vi "Handle Request.vi"(8 "error in (no error)":errorcluster, 9 "Payload":string, 10 "Method":string, 11 "Child Class in":refnum<class "Instrument.lvclass">) -> (0 "error out":errorcluster, 2 "Response":string, 3 "Child Class out":refnum<class "Instrument.lvclass">)   [LabVIEW 2017, in "Instrument.lvlib" / "Instrument.lvclass"]
uses:
  Instrument.lvclass
  <vilib>/TSS/ACRObat Test Framework/Classes/Base Objects/Acrobat Base Object/Acrobat Base Object/Acrobat Base Object.lvclass
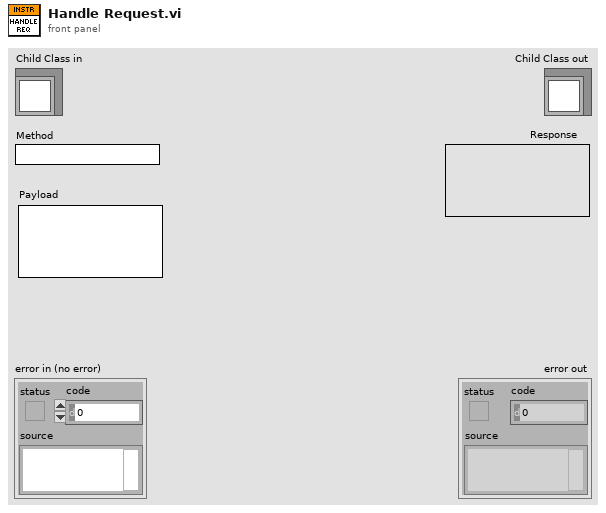
[diagram p1: front panel]
types:
  T1 = cluster{"Self-Test Result Code":i32, "Self-Test Result Message":string}
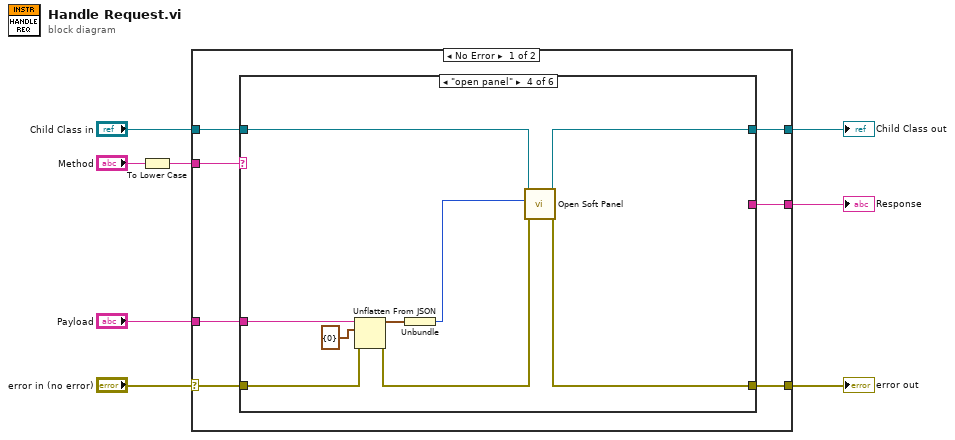
[diagram p0: block diagram]
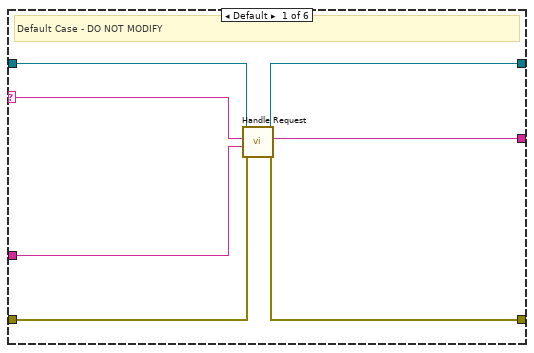
[diagram p2: hidden frame]
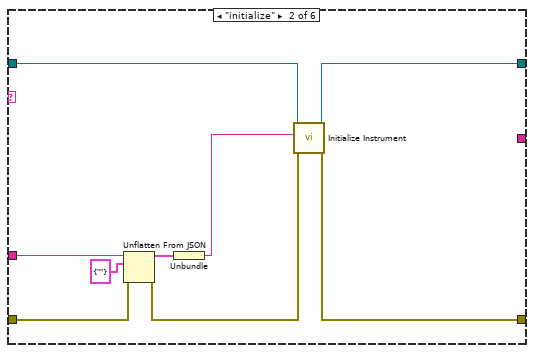
[diagram p3: hidden frame]
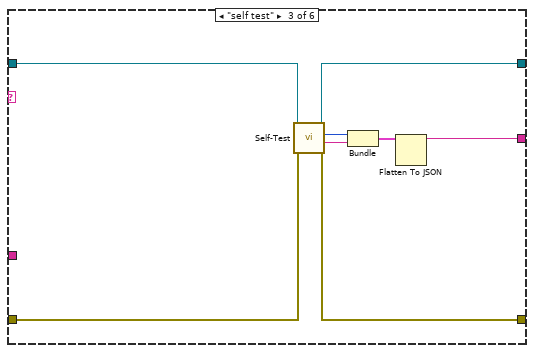
[diagram p4: hidden frame]
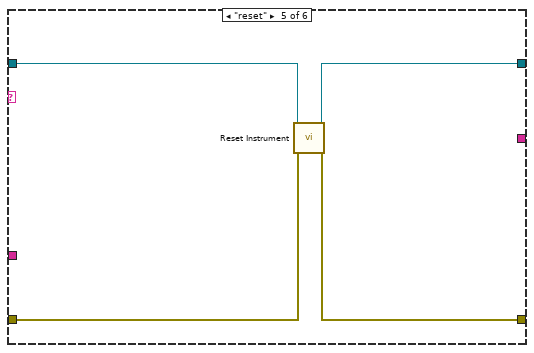
[diagram p5: hidden frame]
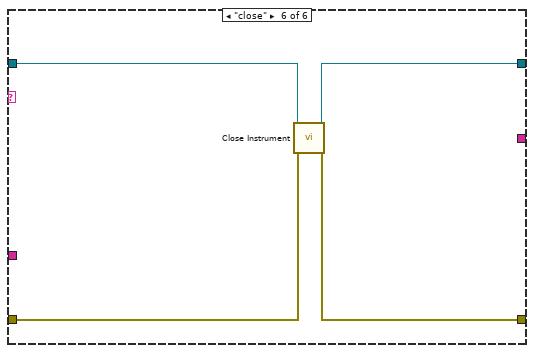
[diagram p6: hidden frame]
diagram:
  n1 = To Lower Case(string="Method") -> (all lower case string=w8:string)
  n2 = case shown="No Error" "error in (no error)" {
    selector: "error in (no error)" -> [w15 w58]
    tunnel: [w14 w58] -> w1
    tunnel: [w11 w57] -> w3
    tunnel: "Child Class in" -> [w12 w57]
    tunnel: w8 -> [w13 _]
    tunnel: "Payload" -> [w9 _]
    tunnel: [w10 _] -> w2
    frame No Error {
      n3 = case shown="\"open panel\"" w13 {
        selector: w13 -> [w17 _ _ _ _ _]
        tunnel: w15 -> [w19 w27 w38 w47 w50 w54]
        tunnel: [w20 w29 w37 w41 w49 w53] -> w14
        tunnel: w12 -> [w22 w31 w39 w44 w52 w56]
        tunnel: [w21 w30 w36 w43 w51 w55] -> w11
        tunnel: [w18 _ w32 _ _ _] -> w10
        tunnel: w9 -> [w16 w28 _ w48 _ _]
        frame Default {
          # "Default Case - DO NOT MODIFY"
          n4 = call-parent "Handle Request.vi"("error in (no error)"=w19, "Payload"=w16, "Method"=w17, "Child Class in"=w22) -> ("error out"=w20:errorcluster, "Response"=w18:string, "Child Class out"=w21:refnum<class "Instrument.lvclass">)  [unwired: 5 in]
        }
        frame "initialize" {
          n5 = Unflatten From JSON(JSON string=w28, type and defaults=cluster{"Instrument Address":string} {"Instrument Address"=""}, error in (no error)=w27) -> (value=w24:cluster{"Instrument Address":string}, error out=w26:errorcluster)  [unwired: 4 in]
          n6 = Unbundle(w24) -> ("Instrument Address"=w23:string)
          n7 = call-dynamic "Initialize Instrument.vi"("error in (no error)"=w26, "Instrument Address"=w23, "Instrument in"=w31) -> ("error out"=w29:errorcluster, "Instrument out"=w30:refnum<class "Instrument.lvclass">)  [unwired: 7 in]
        }
        frame "self test" {
          n8 = call-dynamic "Self-Test.vi"("error in (no error)"=w38, "Instrument in"=w39) -> ("error out"=w37:errorcluster, "Self-Test Result Message"=w34:string, "Self-Test Result Code"=w35:i32, "Instrument out"=w36:refnum<class "Instrument.lvclass">)  [unwired: 6 in]
          n9 = Bundle("Self-Test Result Code"=w35, "Self-Test Result Message"=w34) -> (w33:T1)  [unwired: 1 in]
          n10 = Flatten To JSON(anything=w33) -> (JSON string=w32:string)  [unwired: 2 in, 1 out]
        }
        frame "open panel" {
          n11 = Unflatten From JSON(JSON string=w48, type and defaults=cluster{"SubPanel Ref":u32} {"SubPanel Ref"=0}, error in (no error)=w47) -> (value=w45:cluster{"SubPanel Ref":u32}, error out=w42:errorcluster)  [unwired: 4 in]
          n12 = Unbundle(w45) -> ("SubPanel Ref"=w40:u32)
          n13 = call-dynamic "Open Soft Panel.vi"("error in (no error)"=w42, "SubPanel Ref"=w40, "Instrument in"=w44) -> ("error out"=w41:errorcluster, "Instrument out"=w43:refnum<class "Instrument.lvclass">)  [unwired: 7 in]
        }
        frame "reset" {
          n14 = call-dynamic "Reset Instrument.vi"("error in (no error)"=w50, "Instrument in"=w52) -> ("error out"=w49:errorcluster, "Instrument out"=w51:refnum<class "Instrument.lvclass">)  [unwired: 8 in]
        }
        frame "close" {
          n15 = call-dynamic "Close Instrument.vi"("error in (no error)"=w54, "Instrument in"=w56) -> ("error out"=w53:errorcluster, "Instrument out"=w55:refnum<class "Instrument.lvclass">)  [unwired: 8 in]
        }
      }
    }
    frame Error {
    }
  }
  "error out" <- w1
  "Child Class out" <- w3
  "Response" <- w2
